vi "accessModeToString.vi"(11 "selection":T1) -> (3 "String":string)   [LabVIEW 2020]
uses:
  <vilib>/variable/tagger/mndui/offlineBrowse/MND_browseElementRights.ctl
panel:
  in  "Access Rights Descriptions":string[](array[string])=["None", "Read", "Write", "Read and Write"]
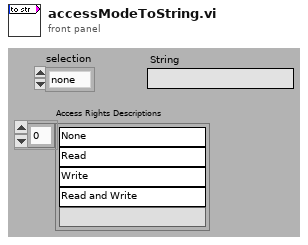
[diagram p1: front panel]
types:
  T1 = typedef "MND_browseElementRights.ctl" = enum16{"none", "read", "write", "read and write"}
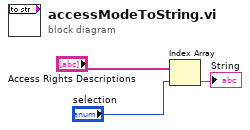
[diagram p0: block diagram]
diagram:
  n1 = Index Array(array="Access Rights Descriptions", index="selection") -> (element=→"String":string)
